vi "Tournament Selection.vi"(8 "error in (no error)":errorcluster, 10 "Tournament Size":i32, 11 "GA.lvclass In":refnum<class "GA.lvclass">) -> (0 "error out":errorcluster, 3 "GA.lvclass Out":refnum<class "GA.lvclass">)   [LabVIEW 2013, in "GA.lvclass"]
uses:
  GA.lvclass
  GA.lvclass/GA.ctl
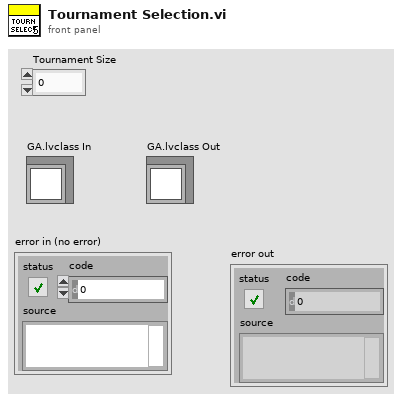
[diagram p1: front panel]
types:
  T1 = typedef "Solution_GA.ctl" = cluster{"Schedule":u16[], "Fitness":u16, "Fitness Valid?":bool}
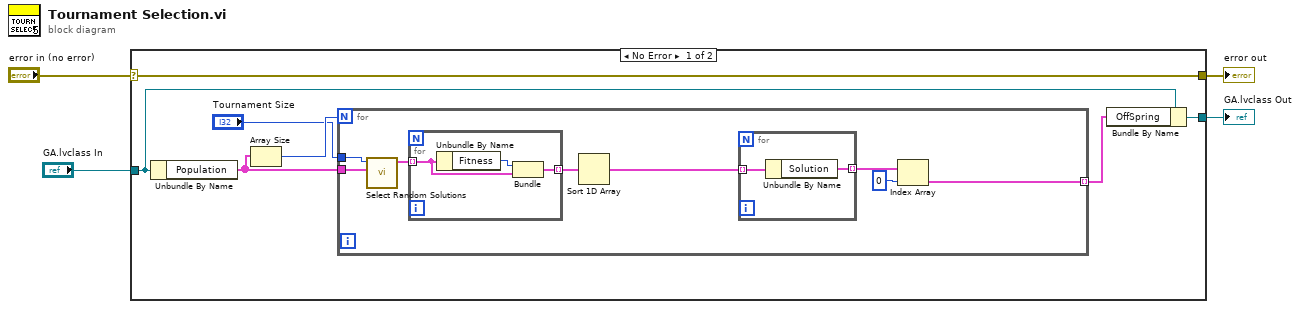
[diagram p0: block diagram]
diagram:
  n1 = case shown="No Error" "error in (no error)" {
    selector: "error in (no error)" -> [w9 w26]
    tunnel: [w9 w26] -> w3
    tunnel: "GA.lvclass In" -> [w6 w25]
    tunnel: [w7 w25] -> w1
    frame No Error {
      n2 = Unbundle By Name(w6) -> ("Population"=w5:T1[])
      n3 = Array Size(array=w5) -> (size(s)=w11:i32)
      n4 = for {
        N: w11 -> [_]
        tunnel: w5 -> [w19]
        tunnel: "Tournament Size" -> [w14]
        tunnel: [w13] -> w8 mode=indexing
        n5 = call "Select Random Solutions.vi"("Population"=w19, "Tournament Size"=w14) -> ("Selected Solutions"=w18:T1[])  [unwired: 9 in]
        n6 = for {
          tunnel: w18 -> [w23] mode=indexing
          tunnel: [w22] -> w17 mode=indexing
          n7 = Unbundle By Name(w23) -> ("Fitness"=w24:u16)
          n8 = Bundle("Fitness"=w24, "Solution"=w23) -> (w22:cluster{"Fitness":u16, "Solution":T1})  [unwired: 1 in]
        }
        n9 = Sort 1D Array(array=w17) -> (sorted array=w12:cluster{"Fitness":u16, "Solution":T1}[])
        n10 = for {
          tunnel: w12 -> [w21] mode=indexing
          tunnel: [w20] -> w16 mode=indexing
          n11 = Unbundle By Name(w21) -> ("Solution"=w20:T1)
        }
        n12 = Index Array(array=w16, index=0) -> (element=w13:T1)
      }
      n13 = Bundle By Name(cluster=w6, "OffSpring"=w8) -> (w7:refnum<class "GA.lvclass">)
    }
    frame Error {
    }
  }
  "error out" <- w3
  "GA.lvclass Out" <- w1
